vi "LDT Parse XML DEC.vi"(8 "error in (no error)":errorcluster, 11 "XML Dec":string="        <hours>12</hours>\n        <minutesTime>10</minutesTime>\n        <secondsTime>35.34</secondsTime>\n") -> (0 "error out":errorcluster, 2 "DEC string":string, 3 "Position.DEC":dbl)   [LabVIEW 2022 SP3, in "LDT Telescope.lvclass"]
uses:
  LDT Telescope.lvclass
  Telescope.lvclass
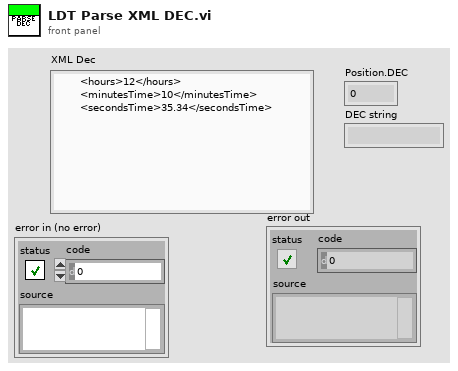
[diagram p1: front panel]
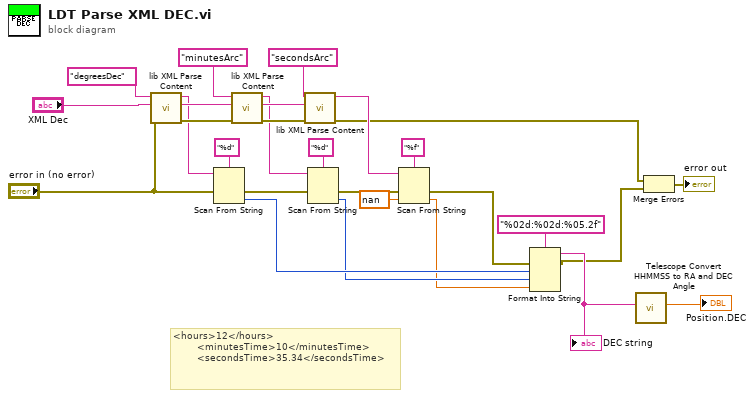
[diagram p0: block diagram]
diagram:
  # "<hours>12</hours>\n        <minutesTime>10</minutesTime>\n        <secondsTime>35.34</secondsTime>"
  n1 = call "lib XML Parse Content.vi"("error in (no error)"="error in (no error)", "XML Line"="XML Dec", "XML Topic"="degreesDec") -> ("error out"=w26:errorcluster, "XML Line dup"=w25:string, "Content"=w20:string)  [unwired: 6 in]
  n2 = Scan From String(format string="%d", input string=w20, error in="error in (no error)") -> (error out=w17:errorcluster, output 1=w10:i32)  [unwired: 2 in, 2 out]
  n3 = call "lib XML Parse Content.vi"("error in (no error)"=w26, "XML Line"=w25, "XML Topic"="minutesArc") -> ("error out"=w21:errorcluster, "XML Line dup"=w23:string, "Content"=w14:string)  [unwired: 6 in]
  n4 = call "lib XML Parse Content.vi"("error in (no error)"=w21, "XML Line"=w23, "XML Topic"="secondsArc") -> ("error out"=w3:errorcluster, "Content"=w13:string)  [unwired: 6 in, 1 out]
  n5 = Scan From String(format string="%d", input string=w14, error in=w17) -> (error out=w12:errorcluster, output 1=w9:i32)  [unwired: 2 in, 2 out]
  n6 = Scan From String(format string="%f", input string=w13, error in=w12, default 1=nan ("default value 1")) -> (error out=w5:errorcluster, output 1=w8:dbl)  [unwired: 1 in, 2 out]
  n7 = Format Into String(format string="%02d:%02d:%05.2f", error in=w5, w10, w9, w8) -> (resulting string=w7:string, error out=w4:errorcluster)  [unwired: 1 in]
  "DEC string" <- w7
  n8 = call "Telescope Convert HHMMSS to RA and DEC Angle.vi"("Dec String"=w7) -> ("DEC"=→"Position.DEC":dbl)  [unwired: 8 in, 2 out]
  n9 = Merge Errors(w3, w4) -> (→"error out":errorcluster)
